vi "User_Console.vi"(8 "error in (no error)":errorcluster) -> (0 "error out":errorcluster)   [LabVIEW 2013]
doc: "The user console. Uses event structure to manage user interactions. Has two way communication, only receives init and shutdown messages. [Covers: UI2]"
uses:
  Requests.ctl
  User_Console_enum.ctl
  Messaging/Msg_Control.ctl
  Error Handler/Error_Control.ctl
panel:
  in  "Requests":T1
  in  "Emergency":bool
  in  "Door Close":bool
  in  "Door Open":bool
  # "[Covers: UI2A]"
  # "First Floor"
  # "[Covers: UI2B]"
  # "Second Floor"
  # "[Covers: UI2B2]"
  # "Make selections Switches"
  # "Third Floor"
  # "Fourth Floor"
  # "[Covers: UI2A1]"
  # "Doors"
  # "[Covers: UI2C]"
  # "[Covers: UI2D]"
  # "Floor Selection"
  # "Elevator Call"
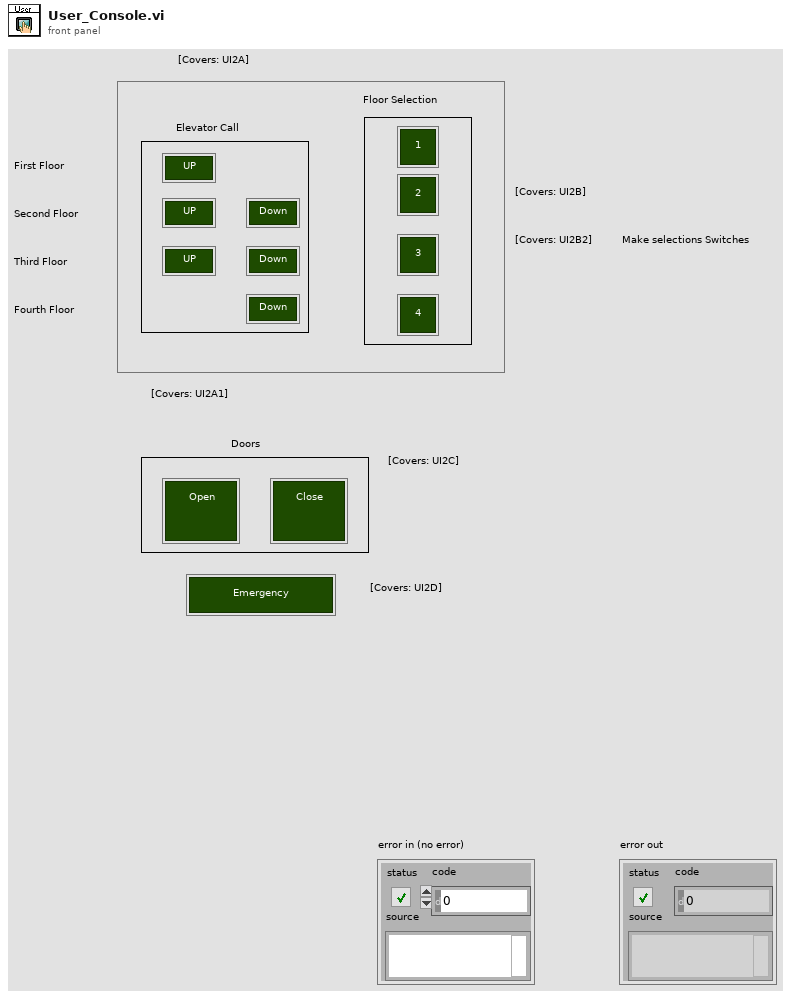
[diagram p1: front panel]
types:
  T1 = typedef "Requests.ctl" = cluster{"1 u":bool, "3 u":bool, "2 u":bool, "2 d":bool, "4 d":bool, "3 d":bool, "1":bool, "2":bool, "3":bool, "4":bool}
  T2 = typedef "Msg_Control.ctl" = enum16{"Init_Msg", "Sent_Inits", "Get_Ref", "Close_Ref"}
  T3 = typedef "User_Console_enum.ctl" = enum16{"Init", "Idle", "Send_Request", "Send_Door", "Send_Emergency", "Receive_Request", "Receive_Door", "Receive_Emergency", "Terminate"}
  T4 = cluster{"queue out":refnum<queue>, "queue out":refnum<queue>, "queue out":refnum<queue>}
  T5 = typedef "Error_Control.ctl" = enum16{"Init", "Console_err", "Process_err", "Sensor_err"}
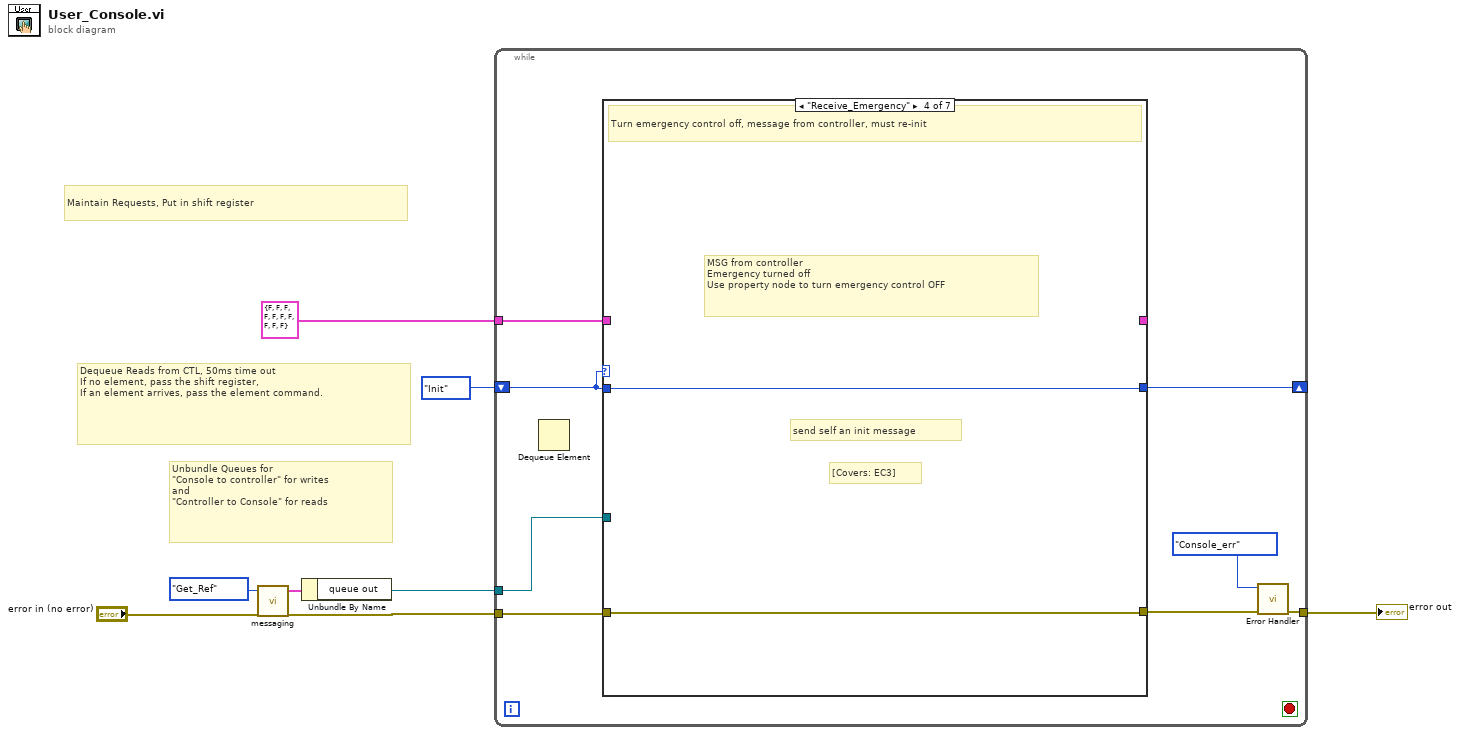
[diagram p0: block diagram]
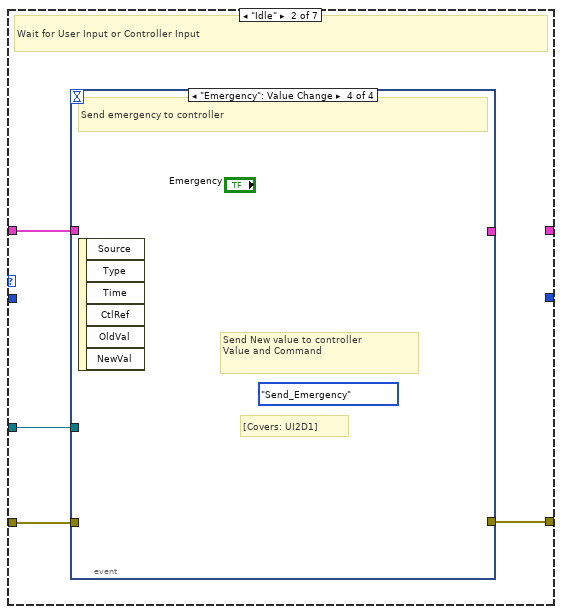
[diagram p3: hidden frame]
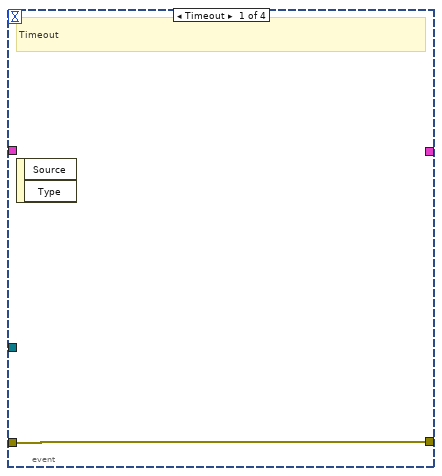
[diagram p4: hidden frame]
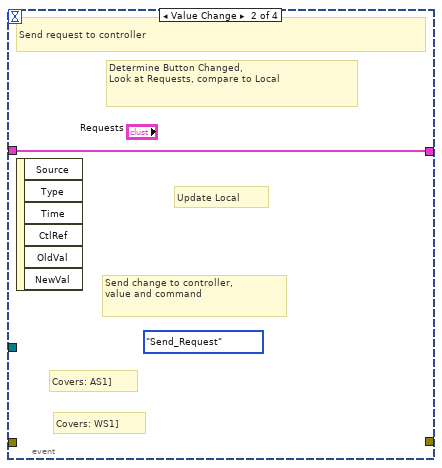
[diagram p5: hidden frame]
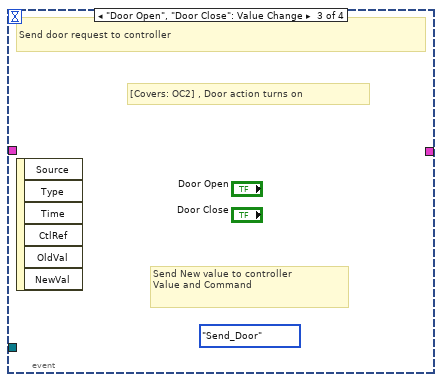
[diagram p6: hidden frame]
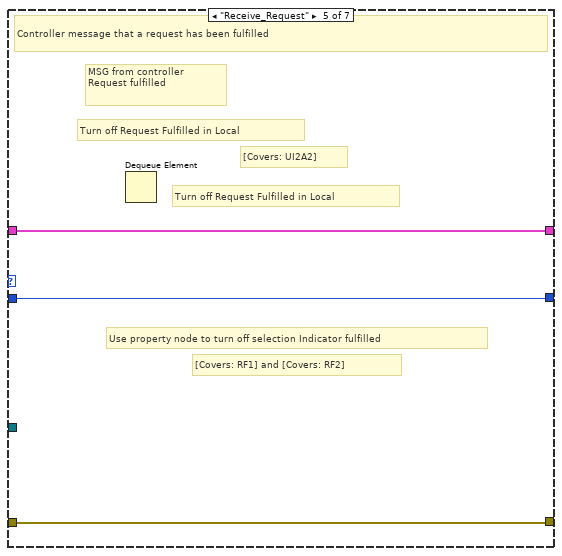
[diagram p8: hidden frame]
diagram:
  # "Dequeue Reads from CTL, 50ms time out\nIf no element, pass the shift register,\nIf an element arrives, pass the element command."
  # "Unbundle Queues for\n\"Console to controller\" for writes\nand\n\"Controller to Console\" for reads"
  # "Maintain Requests, Put in shift register"
  n1 = call "messaging.vi"("error in (no error)"="error in (no error)", "Message_Control"=Msg_Control."Get_Ref") -> ("error out"=w2:errorcluster, "REfs Out"=w4:T4)  [unwired: 8 in]
  n2 = Unbundle By Name(w4) -> ("queue out"=w1:refnum<queue>)
  n3 = while {
    tunnel: [w10] -> w8
    tunnel: T1 {"1 u"=FALSE, "3 u"=FALSE, "2 u"=FALSE, "2 d"=FALSE, "4 d"=FALSE, "3 d"=FALSE, "1"=FALSE, "2"=FALSE, "3"=FALSE, "4"=FALSE} ("Requests") -> [w16]
    tunnel: w2 -> [w15]
    tunnel: w1 -> [w12]
    shift-right: [w13] -> _
    shift-left: User_Console_enum."Init" ("User_Console_Enum") -> [w14]
    stop <- _ stop-if-true
    n4 = Dequeue Element() -> ()  [unwired: 3 in, 4 out]
    n5 = case shown="\"Receive_Emergency\"" w14 {
      tunnel: w16 -> [_ w20 _ _ w29 _ _]
      tunnel: w15 -> [w17 w21 w25 w27 w30 w32 w34]
      tunnel: [w18 _ w26 w28 w31 w33 w35] -> w13
      tunnel: w14 -> [w18 _ w26 w28 w31 w33 w35]
      tunnel: w12 -> [_ w19 _ _ _ _ _]
      tunnel: [w17 w22 w25 w27 w30 w32 w34] -> w11
      tunnel: [_ _ _ _ w29 _ _] -> _
      frame "Init", Default {
        # "Pass the Requests cluster"
        # "Use property nodes to turn all selections to OFF, Open and Close to OFF, \nand the emergency to off.  [Covers: IS3]"
        # "Initialize all controls [Covers: IS1]"
      }
      frame "Idle" {
        # "Wait for User Input or Controller Input"
        n6 = event shown="[3] \"Emergency\": Value Change" {
          selector: _ -> [_ _ _ _]
          dyn-events: _ -> [_ _ _ _]
          timeout: _ -> [_ _ _ _]
          tunnel: [w23 _ _ _] -> w22
          tunnel: w21 -> [w23 _ _ _]
          tunnel: w20 -> [_ w24 _ _]
          tunnel: [_ w24 _ _] -> _
          tunnel: w19 -> [_ _ _ _]
          event Timeout {
            # "Timeout"
            n7 = event-data() -> ()  [unwired: 1 in, 2 out]
          }
          event Value Change {
            (unwired) User_Console_enum."Send_Request" ("User_Console_Enum")
            # "Covers: WS1]"
            # "Covers: AS1]"
            # "Update Local"
            # "Send change to controller, \nvalue and command"
            # "Determine Button Changed,\nLook at Requests, compare to Local"
            # "Send request to controller"
            n8 = event-data() -> ()  [unwired: 1 in, 6 out]
          }
          event "Door Open", "Door Close": Value Change {
            (unwired) User_Console_enum."Send_Door" ("User_Console_Enum")
            # "[Covers: OC2] , Door action turns on"
            # "Send New value to controller\nValue and Command"
            # "Send door request to controller"
            n9 = event-data() -> ()  [unwired: 1 in, 6 out]
          }
          event "Emergency": Value Change {
            (unwired) User_Console_enum."Send_Emergency" ("User_Console_Enum")
            # "[Covers: UI2D1]"
            # "Send New value to controller\nValue and Command"
            # "Send emergency to controller"
            n10 = event-data() -> ()  [unwired: 1 in, 6 out]
          }
        }
      }
      frame "Receive_Door" {
        # "[Covers: UI2C3]"
        # "Message from controller\nDisable Doors"
        # "Command from Controller for Door closing"
      }
      frame "Receive_Emergency" {
        # "send self an init message"
        # "[Covers: EC3]"
        # "MSG from controller\nEmergency turned off\nUse property node to turn emergency control OFF"
        # "Turn emergency control off, message from controller, must re-init"
      }
      frame "Receive_Request" {
        # "[Covers: UI2A2]"
        # "Use property node to turn off selection Indicator fulfilled"
        # "[Covers: RF1] and [Covers: RF2]"
        # "Turn off Request Fulfilled in Local"
        # "Turn off Request Fulfilled in Local"
        # "MSG from controller\nRequest fulfilled"
        # "Controller message that a request has been fulfilled"
        n11 = Dequeue Element() -> ()  [unwired: 3 in, 4 out]
      }
      frame "Send_Request".."Send_Emergency" {
        # "Not Used"
        # "These commands not used,"
      }
      frame "Terminate" {
        # "[Covers: TS2]"
        # "Shut down loop, Send TRUE to loop condition"
        # "Disable All Controls\n[Covers: TS1]"
        # "Disable Controls, end loop"
      }
    }
    n12 = call "Error Handler.vi"("error in (no error)"=w11, "Error_Control"=Error_Control."Console_err") -> ("error out"=w10:errorcluster)  [unwired: 9 in]
  }
  "error out" <- w8
